vi "Example_Simple Acquire one graph.vi"() -> ()   [LabVIEW 2015, in "G 5.lvlib"]
uses:
  G 5.lvlib
  <vilib>/Utility/file.llb/Write To Spreadsheet File (DBL).vi
panel:
  out "Array":waveform(dbl)[](array[waveform])
  in  "Display Duration [sec]":dbl=10.0
  in  "Acquisition Rate [Hz]":i16(ring)=2000 items=["10"=10, "15"=15, "20"=20, "25"=25, "30"=30, "40"=40, "45"=45, "50"=50, "60"=60, "75"=75, "80"=80, "90"=90, "100"=100, "120"=120, "125"=125, "150"=150, "180"=180, "200"=200, "225"=225, "240"=240, "250"=250, "300"=300, "360"=360, "400"=400, "450"=450, "500"=500, "600"=600, "800"=800, "900"=900, "1000"=1000, "1200"=1200, "1500"=1500, "1800"=1800, "2000"=2000]
  in  "Save Data":bool
  in  "Start Acquisition":bool
  in  "stop":bool
  in  "ZERO":bool
  in  "Gen 5":i32=1 min=1 step=1
  in  "CAPTURE":bool
  out "STATUS":bool=TRUE
  in  "Channel":i32=3
  in  "Value":dbl=5.0
  in  "Time [sec]":dbl=0.5 step=0.1 format="%.2g"
  in  "Gen 5 Displayed 1":i64=1
  # "TRIGGER CONTROL"
  # "ACQUISITION SETUP"
  # "ACQUISITION CONTROL"
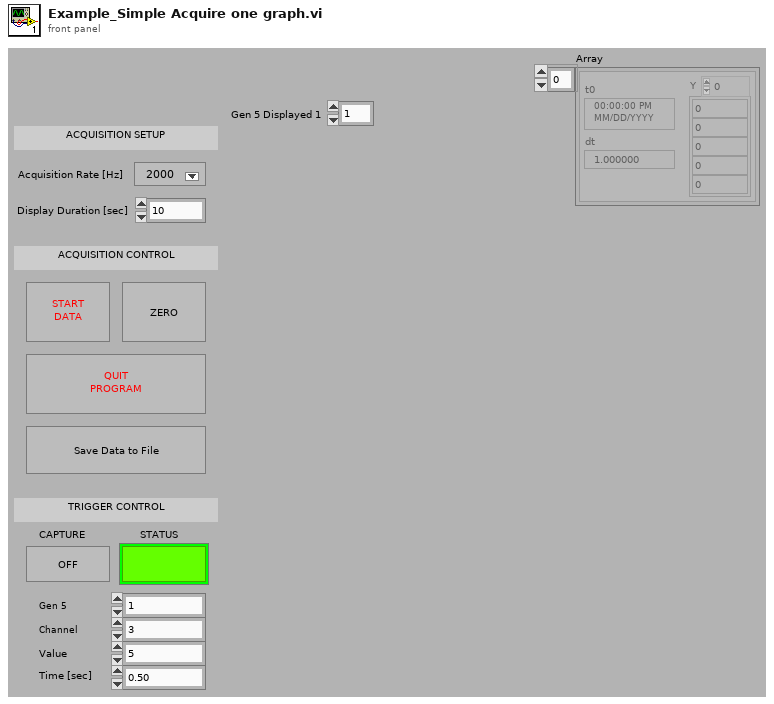
[diagram p1: front panel]
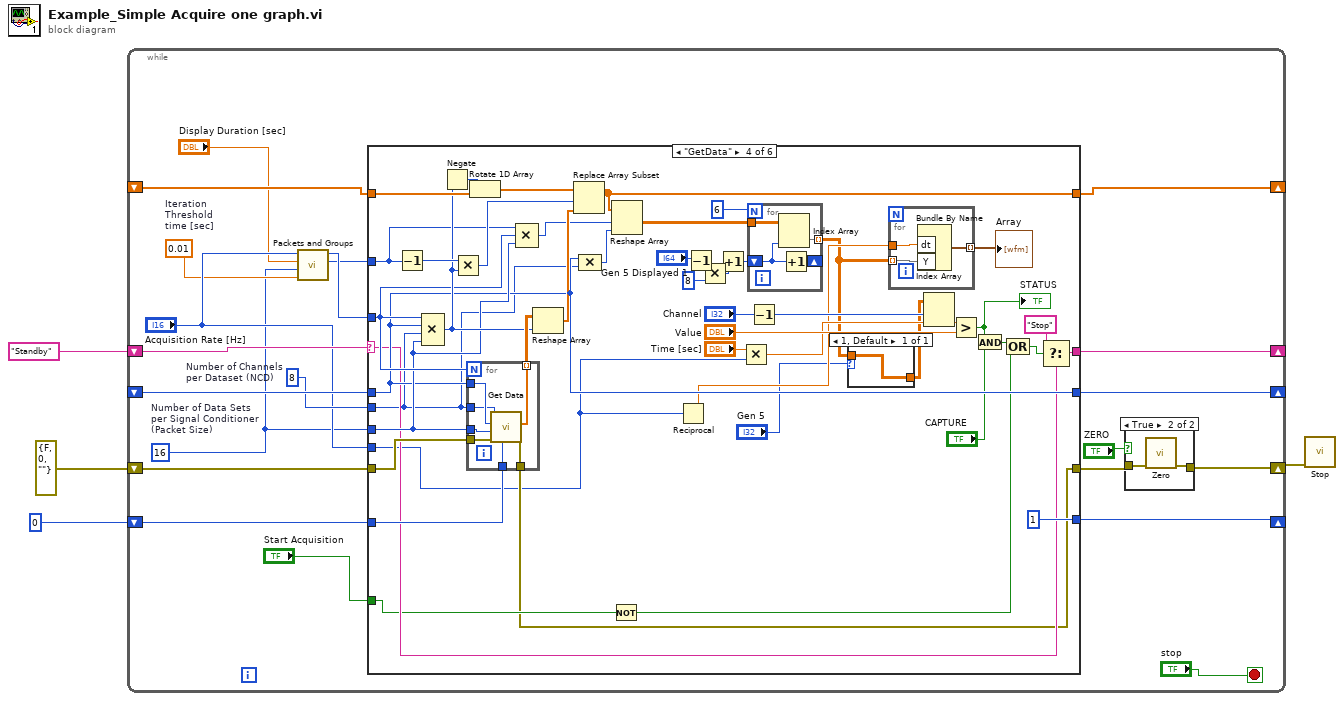
[diagram p0: block diagram]
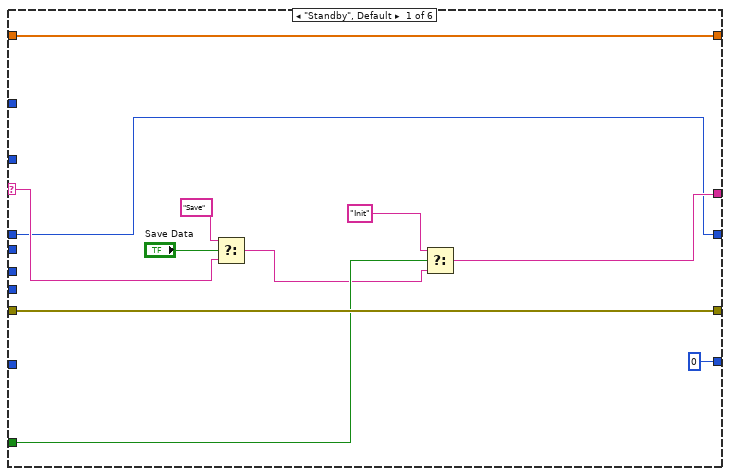
[diagram p3: hidden frame]
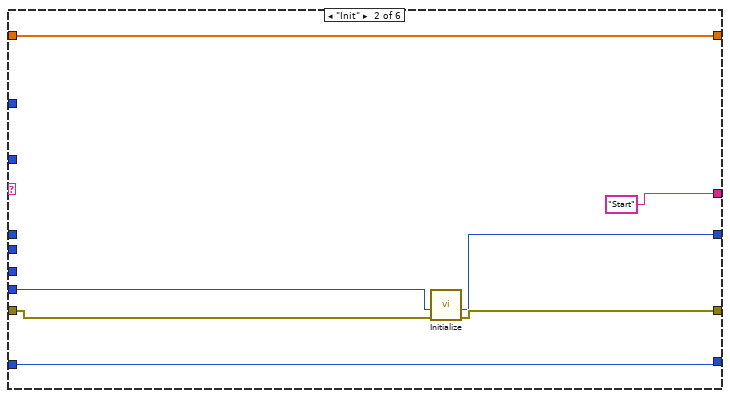
[diagram p4: hidden frame]
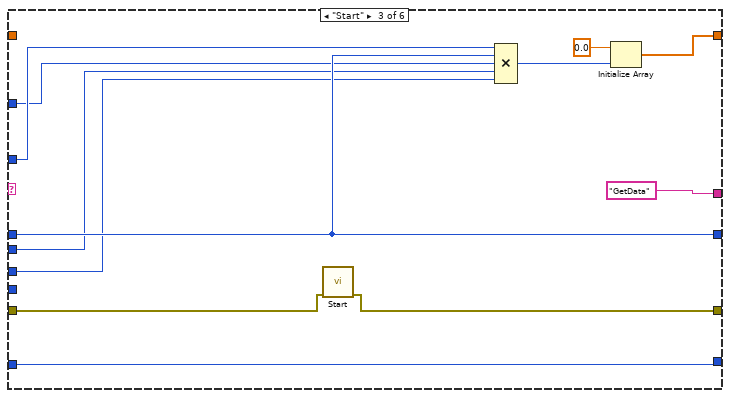
[diagram p5: hidden frame]
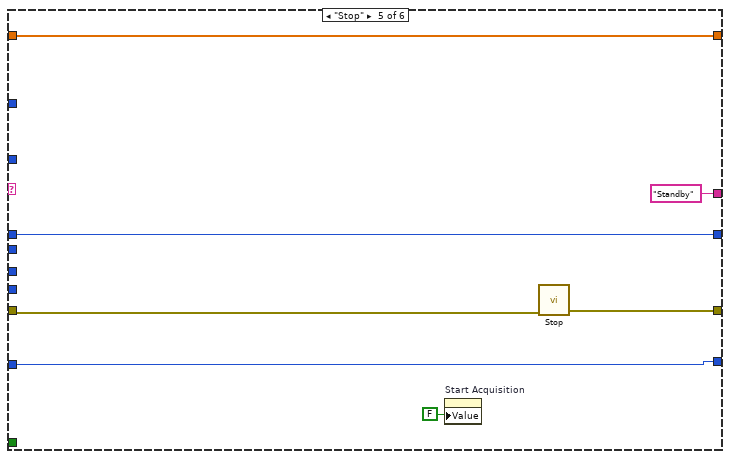
[diagram p6: hidden frame]
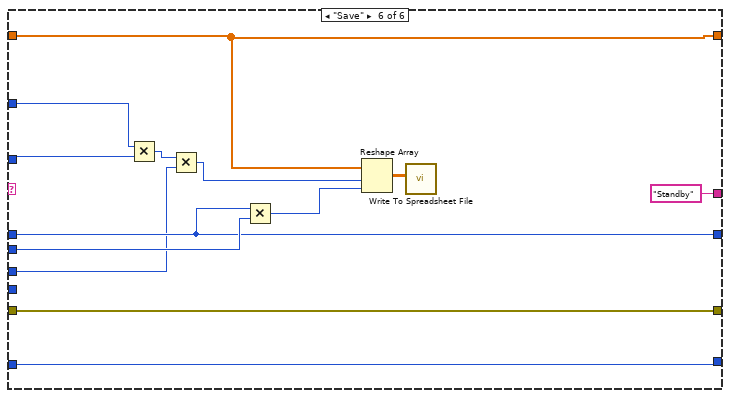
[diagram p7: hidden frame]
diagram:
  n1 = while {
    shift-right: [w20] -> _
    shift-left: "Standby" -> [w25]
    shift-right: [w23] -> w1
    shift-left: errorcluster {"status"=FALSE, "code"=0, "source"=""} ("error out") -> [w22]
    shift-right: [w19] -> _
    shift-left: _ -> [w18]
    shift-right: [w16] -> _
    shift-left: 0 -> [w17]
    shift-right: [w13] -> _
    shift-left: _ -> [w14]
    stop <- "stop" stop-if-true
    w9 = 0.01  # Iteration  Threshold  time [sec]
    w15 = 8  # Number of Channels per Dataset (NCD)
    w6 = 16  # Number of Data Sets  per Signal Conditioner (Packet Size)
    n2 = call "Packets and Groups.vi"("Iteration Treshold Time [sec]"=w9, "Packet Size"=w6, "Duration [sec]"="Display Duration [sec]", "Acquisition Rate"="Acquisition Rate [Hz]") -> ("GROUPS"=w7:i32, "PACKETS"=w8:i32)  [unwired: 4 in, 2 out]
    n3 = case shown="\"GetData\"" w25 {
      selector: w25 -> [w32 _ _ w76 _ _]
      tunnel: w22 -> [w39 w46 w57 w104 w127 w138]
      tunnel: [w39 w45 w58 w70 w128 w138] -> w21
      tunnel: [w38 "Start" "GetData" w75 "Standby" "Standby"] -> w20
      tunnel: "Acquisition Rate [Hz]" -> [_ w43 _ w63 _ _]
      tunnel: [w29 w42 w51 w84 w125 w134] -> w19
      tunnel: w18 -> [w29 _ w51 w84 w125 w134]
      tunnel: w17 -> [_ w41 w47 w106 w124 w137]
      tunnel: [0 w41 w47 1 w124 w137] -> w16
      tunnel: w8 -> [_ _ w52 w91 _ w129]
      tunnel: w6 -> [_ _ w48 w90 _ w131]
      tunnel: w15 -> [_ _ w49 w72 _ w135]
      tunnel: w14 -> [w35 w40 _ w102 w123 w140]
      tunnel: w7 -> [_ _ w50 w92 _ w130]
      tunnel: [w35 w40 w54 w95 w123 w140] -> w13
      tunnel: "Start Acquisition" -> [w34 _ _ w73 _ _]
      frame "Standby", Default {
        n4 = Select(t="Save", s="Save Data", f=w32) -> (s? t:f=w31:string)
        n5 = Select(t="Init", s=w34, f=w31) -> (s? t:f=w38:string)
      }
      frame "Init" {
        n6 = call "Initialize.vi"("error in (no error)"=w46, "Acquisition Rate"=w43) -> ("error out"=w45:errorcluster, "Device Count"=w42:i32)  [unwired: 8 in]
      }
      frame "Start" {
        n7 = call "Start.vi"("error in (no error)"=w57) -> ("error out"=w58:errorcluster)  [unwired: 10 in]
        n8 = Compound Arithmetic op=MULTIPLY(w52, w51, w50, w49, w48) -> (w53:i32)
        n9 = Initialize Array(0.0 ("element"), w53) -> (w54:dbl[])
      }
      frame "GetData" {
        n10 = Decrement(x=w92) -> (x-1=w98:i32)
        n11 = Compound Arithmetic op=MULTIPLY(w91, w84, w72, w90) -> (w97:i32)
        n12 = Negate(x=w97) -> (-x=w101:i32)
        n13 = Multiply(x=w98, y=w97) -> (x*y=w96:i32)
        n14 = for {
          N: w91 -> [_]
          tunnel: w106 -> [w121]
          tunnel: [w117] -> w70
          tunnel: w84 -> [w118]
          tunnel: w104 -> [w120]
          tunnel: [w119] -> w103 mode=indexing
          tunnel: w90 -> [w116]
          tunnel: w72 -> [w115]
          n15 = call "Get Data.vi"("Iteration"=w121, "error in"=w120, "N_DataSets\nper Gen5"=w116, "Device Count"=w118, "N_Channels\nper Dataset (NCD)"=w115) -> ("error out"=w117:errorcluster, "Data out"=w119:sgl[])  [unwired: 5 in]
        }
        n16 = Rotate 1D Array(1:w102, 2:w101) -> (0:w100:dbl[])
        n17 = Compound Arithmetic op=MULTIPLY(w92, w91, w90) -> (w94:i32)
        n18 = Reshape Array(w103, w97) -> (w99:sgl[])
        n19 = Replace Array Subset(array=w100, new element=w99, index=w96) -> (w95:dbl[])
        n20 = Compound Arithmetic op=MULTIPLY(w84, w72) -> (w93:i32)
        n21 = Not(x=w73) -> (.not. x?=w65:bool)
        n22 = Reshape Array(w95, w94, w93) -> (w68:dbl[][])
        n23 = Reciprocal(x=w63) -> (1/x=w69:dbl)
        n24 = Decrement(x="Gen 5 Displayed 1") -> (x-1=w87:i64)
        n25 = Multiply(x=w87, y=i64 8) -> (x*y=w85:i64)
        n26 = Increment(x=w85) -> (x+1=w67:i64)
        n27 = Multiply(x="Time [sec]", y=w63) -> (x*y=w71:dbl)
        n28 = for {
          N: 6 -> [_]
          tunnel: w68 -> [w114]
          tunnel: [w113] -> w61 mode=indexing
          shift-right: [w112] -> _
          shift-left: w67 -> [w111]
          n29 = Index Array(array=w114, index (col)=w111) -> (element=w113:dbl[])  [unwired: 1 in]
          n30 = Increment(x=w111) -> (x+1=w112:i64)
        }
        n31 = Decrement(x="Channel") -> (x-1=w80:i32)
        n32 = case shown="1, Default" "Gen 5" {
          tunnel: w61 -> [w107]
          tunnel: [w107] -> w60
          frame 1, Default {
          }
        }
        n33 = for {
          tunnel: [w110] -> w59 mode=indexing
          tunnel: w61 -> [w109] mode=indexing
          tunnel: w69 -> [w108]
          n34 = Bundle By Name("dt"=w108, "Y"=w109) -> (w110:waveform(dbl))  [unwired: 1 in]
        }
        "Array" <- w59
        n35 = Index Array(array=w60, index (row)=w80, index (col)=w71) -> (element=w82:dbl)
        n36 = Greater?(x=w82, y="Value") -> (0:w77:bool)
        "STATUS" <- w77
        n37 = And(x=w77, y="CAPTURE") -> (x .and. y?=w66:bool)
        n38 = Compound Arithmetic op=OR(w66, w65) -> (w64:bool)
        n39 = Select(t="Stop", s=w64, f=w76) -> (s? t:f=w75:string)
      }
      frame "Stop" {
        n40 = property on="Start Acquisition" class="Bool (strict)"("Value"=FALSE ("Start Acquisition")) -> ()  [unwired: 2 in, 2 out]
        n41 = call "Stop.vi"("error in (no error)"=w127) -> ("error out"=w128:errorcluster)  [unwired: 10 in]
      }
      frame "Save" {
        n42 = Multiply(x=w130, y=w129) -> (x*y=w132:i32)
        n43 = Multiply(x=w132, y=w131) -> (x*y=w133:i32)
        n44 = Multiply(x=w134, y=w135) -> (x*y=w136:i32)
        n45 = Reshape Array(w140, w133, w136) -> (w141:dbl[][])
        n46 = call-poly <vilib>:"Write To Spreadsheet File.vi"("2D data"=w141) -> ()  [unwired: 7 in, 1 out]
      }
    }
    n47 = case shown="True" "ZERO" {
      tunnel: w21 -> [w26 w28]
      tunnel: [w26 w27] -> w23
      frame False {
      }
      frame True {
        n48 = call "Zero.vi"("error in (no error)"=w28) -> ("error out"=w27:errorcluster)  [unwired: 10 in]
      }
    }
  }
  n49 = call "Stop.vi"("error in (no error)"=w1) -> ()  [unwired: 10 in, 1 out]
